vi "run.vi"(8 "error in (no error)":errorcluster, 11 "GenericLightSource in":refnum<class "GenericLightSource.lvclass">) -> (0 "error out":errorcluster, 3 "GenericLightSource out":refnum<class "GenericLightSource.lvclass">)   [LabVIEW 2010]
uses:
  main/labview_source/main/main_statechart.lvsc/Trigger.ctl
  main/labview_source/main/main_statechart.lvsc
  main/labview_source/type_definitions/classes/GenericStage/trigger_enum.ctl
  main/labview_source/type_definitions/classes/GenericStage/GenericStage.lvclass
  GenericLightSource.lvclass
panel:
  # "Functionality not available..."
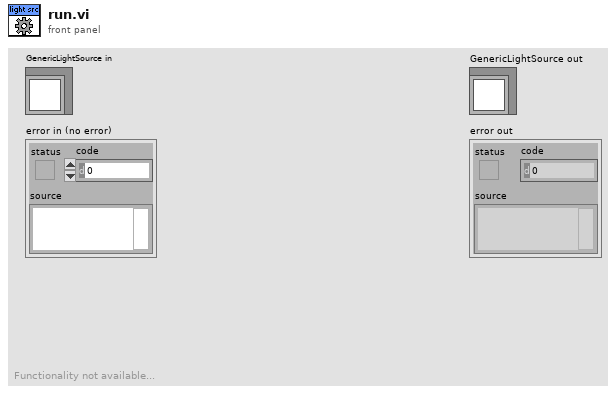
[diagram p1: front panel]
types:
  T1 = typedef "main_statechart.lvsc/Trigger.ctl" = enum16{"NULL", "initialise", "terminate", "start", "stop", "experiment controller ready", "experiment controller missing", "scan mode ready", "scan mode missing", "scan head ready", "scan head missing", "DAQ ready", "DAQ missing", "image assembler ready", "image assembler missing", "data collection ready", "data collection missing", "display ready", "display missing", "analyser ready", "analyser missing", "stage ready", "stage missing", "stimulator ready", "stimulator missing", "instrument ready", "instrument missing", "change objective", "change imagingMode", "change experimentController", "save notebook", "started saving", "finished saving"}
  T2 = typedef "GenericStage.lvclass/trigger_enum.ctl" = enum16{"NULL", "initialise", "terminate", "move", "update position", "set origin", "return to origin"}
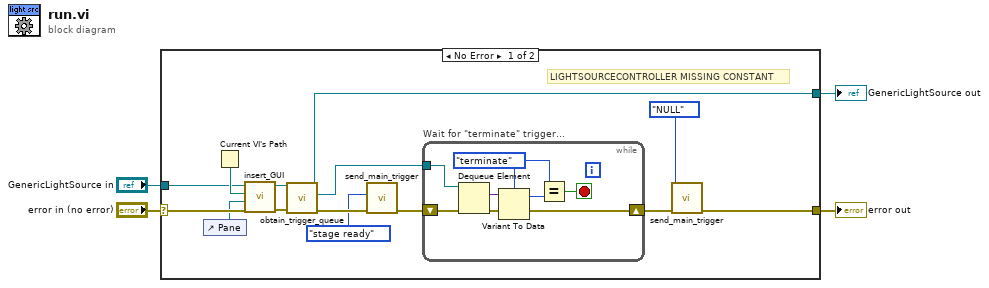
[diagram p0: block diagram]
diagram:
  n1 = case shown="No Error" "error in (no error)" {
    selector: "error in (no error)" -> [w10 w28]
    tunnel: [w9 w28] -> w1
    tunnel: [w7 w27] -> w2
    tunnel: "GenericLightSource in" -> [w8 w27]
    frame No Error {
      # "LIGHTSOURCECONTROLLER MISSING CONSTANT"
      n2 = control-ref of="Pane"() -> (w5:refnum<vi>)
      n3 = Current VI's Path() -> (path=w18:path)
      n4 = call-dynamic "insert_GUI.vi"("error in (no error)"=w10, "Pane"=w5, "VI path"=w18, "GenericComponent in"=w8) -> ("error out"=w17:errorcluster, "GenericComponent out"=w16:refnum<class "GenericLightSource.lvclass">)  [unwired: 6 in]
      n5 = call-dynamic "obtain_trigger_queue.vi"("error in (no error)"=w17, "GenericPlugin in"=w16) -> ("error out"=w14:errorcluster, "trigger queue"=w13:refnum<queue>, "GenericPlugin out"=w7:refnum<class "GenericLightSource.lvclass">)  [unwired: 7 in]
      n6 = call "send_main_trigger.vi"("error in (no error)"=w14, "trigger"=Trigger."stage ready") -> ("error out"=w15:errorcluster)  [unwired: 9 in]
      n7 = while "Wait for \"terminate\" trigger..." {
        shift-right: [w19] -> w11
        shift-left: w15 -> [w26]
        tunnel: w13 -> [w25]
        stop <- w24 stop-if-true
        w20 = trigger_enum."terminate" ("trigger")
        n8 = Dequeue Element(queue=w25, error in (no error)=w26) -> (element=w22:variant, error out=w23:errorcluster)  [unwired: 1 in, 2 out]
        n9 = Variant To Data(error in=w23, Variant=w22, type=w20) -> (error out=w19:errorcluster, data=w21:T2)
        n10 = Equal?(x=w20, y=w21) -> (x = y?=w24:bool)
      }
      n11 = call "send_main_trigger.vi"("error in (no error)"=w11, "trigger"=Trigger."NULL") -> ("error out"=w9:errorcluster)  [unwired: 9 in]
    }
    frame Error {
    }
  }
  "error out" <- w1
  "GenericLightSource out" <- w2
